vi "DoSomething.vi"(9 "Cluster":T1, 10 "String":string, 11 "Numeric":dbl) -> (3 "Cluster 2":T1)   [LabVIEW 2010]
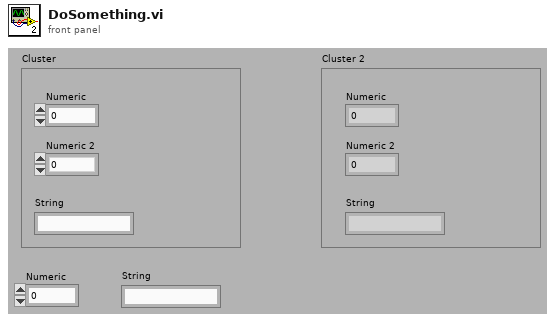
[diagram p1: front panel]
types:
  T1 = cluster{"Numeric":dbl, "Numeric 2":dbl, "String":string}
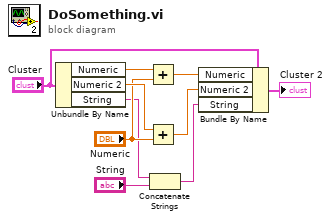
[diagram p0: block diagram]
diagram:
  n1 = Unbundle By Name("Cluster") -> ("Numeric"=w10:dbl, "Numeric 2"=w9:dbl, "String"=w3:string)
  n2 = Add(x=w10, y="Numeric") -> (x+y=w5:dbl)
  n3 = Add(x=w9, y="Numeric") -> (x+y=w4:dbl)
  n4 = Concatenate Strings(w3, "String") -> (w1:string)
  n5 = Bundle By Name(cluster="Cluster", "Numeric"=w5, "Numeric 2"=w4, "String"=w1) -> (→"Cluster 2":T1)
